vi "how to paly.vi"() -> ()   [LabVIEW 2014]
uses:
  airplane.ctl
  nail.ctl
  block.ctl
panel:
  in  "Block":T1
  in  "Block 2":T2
  in  "bird":T3
  in  "OK Button":bool
  # "Press '' SPACE  BAR'' to jump"
  # "skipped over the obstacle"
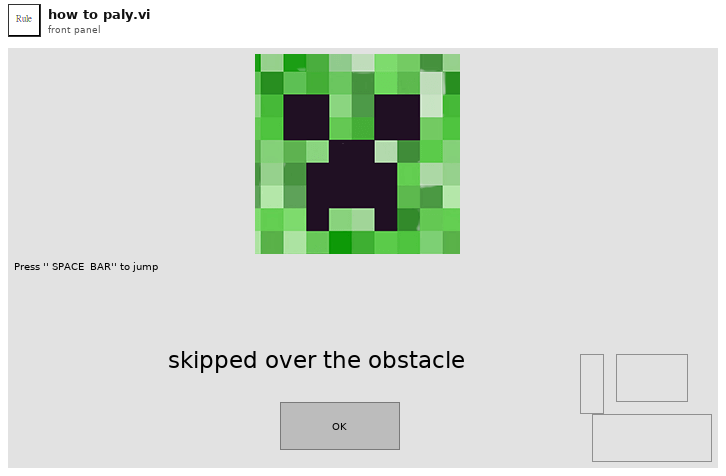
[diagram p1: front panel]
types:
  T1 = typedef "block.ctl" = bool
  T2 = typedef "nail.ctl" = bool
  T3 = typedef "airplane.ctl" = bool
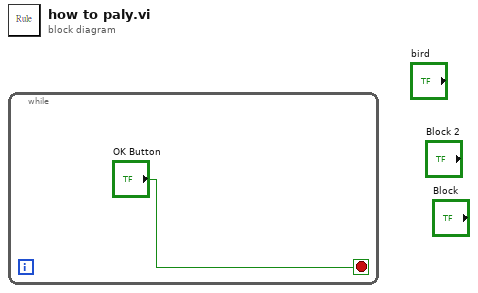
[diagram p0: block diagram]
diagram:
  n1 = while {
    stop <- "OK Button" stop-if-true
  }
